vi "Get DI Camera Info.vi"(11 "info":u32) -> (2 "function return":u32, 3 "info out":u32)   [LabVIEW 2018, in "Copy of Andor SDK.lvlib"]
doc: "EXPNETTYPE unsigned int WINAPI GetDICameraInfo(void * info);"
uses:
  Copy of Andor SDK.lvlib
  <userlib>/Andor SDK/ATMCD32D.dll
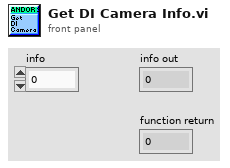
[diagram p1: front panel]
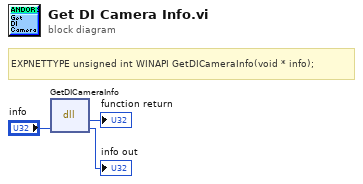
[diagram p0: block diagram]
diagram:
  # "EXPNETTYPE unsigned int WINAPI GetDICameraInfo(void * info);"
  n1 = dll-call lib="C:/Program Files (x86)/National Instruments/LabVIEW 2018/user.lib/Andor SDK/ATMCD32D.*" fn="GetDICameraInfo"("info"="info") -> (→"function return":u32, "info"=→"info out":u32)  [unwired: 3 in, 2 out]
